vi "Teleop.vi"(8 "Driver Command Inputs":T8, 9 "Sensor Inputs":T1, 10 "Match Info":T16={"Autonomous Elapsed Seconds"=0.0, "TeleOp Elapsed Seconds"=0.0, "Disabled Elapsed Seconds"=0.0, "Visited Autonomous"=FALSE, "Visited TeleOp"=FALSE, "Visited Disabled"=FALSE, "Autonomous Settings"={"Autonomous Style"=enum."Independent", "VI Refnum"=refnum}}, 11 "Call Context":T17) -> (2 "Commands":T8, 3 "Sensor Inputs":T1)   [LabVIEW 2012]
doc: "This VI is called for each TeleOp packet received from the DS where the robot is not disabled. It is often used to read from the joysticks and update I/O or to update setpoints for timed control loops. It should complete and return within 20 milliseconds or it may miss DS packets."
uses:
  <vilib>/Rock Robotics/WPI/DriverStation/WPI_DriverStationDerivedRobotMode.ctl
  <vilib>/Rock Robotics/WPI/DriverStation/WPI_DriverStationMatch Info.ctl
  Inputs_All.ctl
  Flywheel/Sensor_Inputs_FlyWheel.ctl
  tankdrive/Input_Sensors_Drive.ctl
  Conveyor/Sensor_Input_Conveyor.ctl
  Conveyor/Sensor_Input_ConveyorV2.ctl
  Turret/Inputs_Sensors_Turret.ctl
  Inputs_Camera.ctl
  Command_Inputs.ctl
  tankdrive/Input_Commands_Drive.ctl
  Conveyor/Input_Command_Conveyor.ctl
  Turret/Inputs_Commands_Turret.ctl
  Bridge Tipper/Inputs_Tipper.ctl
  Dashboard Controls.ctl
  Roller/Input_Commands_Roller.ctl
  Flywheel/Input_Commands_Flywheel.ctl
  Robot Global Data.vi
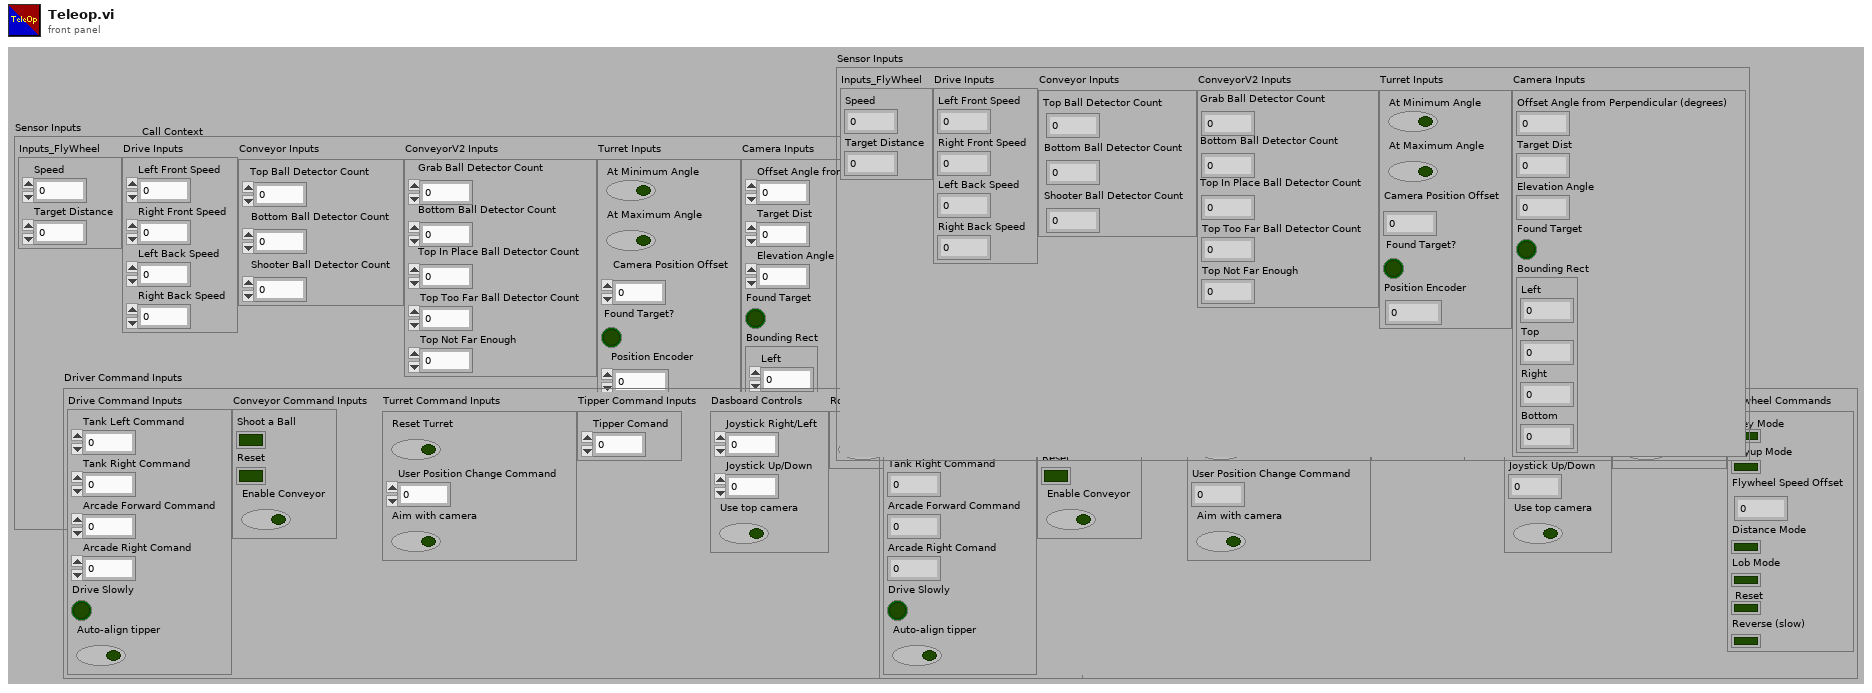
[diagram p1: front panel]
types:
  T1 = typedef "Inputs_All.ctl" = cluster{"Inputs_FlyWheel":T2, "Drive Inputs":T3, "Conveyor Inputs":T4, "ConveyorV2 Inputs":T5, "Turret Inputs":T6, "Camera Inputs":T7}
  T2 = typedef "Sensor_Inputs_FlyWheel.ctl" = cluster{"Speed":dbl, "Target Distance":dbl}
  T3 = typedef "Input_Sensors_Drive.ctl" = cluster{"Left Front Speed":dbl, "Right Front Speed":dbl, "Left Back Speed":dbl, "Right Back Speed":dbl}
  T4 = typedef "Sensor_Input_Conveyor.ctl" = cluster{"Top Ball Detector Count":i32, "Bottom Ball Detector Count":i32, "Shooter Ball Detector Count":i32}
  T5 = typedef "Sensor_Input_ConveyorV2.ctl" = cluster{"Grab Ball Detector Count":i32, "Bottom Ball Detector Count":i32, "Top In Place Ball Detector Count":i32, "Top Too Far Ball Detector Count":i32, "Top Not Far Enough":i32}
  T6 = typedef "Inputs_Sensors_Turret.ctl" = cluster{"At Minimum Angle":bool, "At Maximum Angle":bool, "Camera Position Offset":dbl, "Found Target?":bool, "Position Encoder":dbl}
  T7 = typedef "Inputs_Camera.ctl" = cluster{"Offset Angle from Perpendicular (degrees)":dbl, "Target Dist":dbl, "Elevation Angle":dbl, "Found Target":bool, "Bounding Rect":cluster{"Left":dbl, "Top":dbl, "Right":dbl, "Bottom":dbl}}
  T8 = typedef "Command_Inputs.ctl" = cluster{"Drive Command Inputs":T9, "Conveyor Command Inputs":T10, "Turret Command Inputs":T11, "Tipper Command Inputs":T12, "Dasboard Controls":T13, "Roller Commands":T14, "Flywheel Commands":T15}
  T9 = typedef "Input_Commands_Drive.ctl" = cluster{"Tank Left Command":dbl, "Tank Right Command":dbl, "Arcade Forward Command":dbl, "Arcade Right Comand":dbl, "Drive Slowly":bool, "Auto-align tipper":bool}
  T10 = typedef "Input_Command_Conveyor.ctl" = cluster{"Shoot a Ball":bool, "Reset":bool, "Enable Conveyor":bool}
  T11 = typedef "Inputs_Commands_Turret.ctl" = cluster{"Reset Turret":bool, "User Position Change Command":dbl, "Aim with camera":bool}
  T12 = typedef "Inputs_Tipper.ctl" = cluster{"Tipper Comand":dbl}
  T13 = typedef "Dashboard Controls.ctl" = cluster{"Joystick Right/Left":dbl, "Joystick Up/Down":dbl, "Use top camera":bool}
  T14 = typedef "Input_Commands_Roller.ctl" = cluster{"Enable Front Roller":bool}
  T15 = typedef "Input_Commands_Flywheel.ctl" = cluster{"Key Mode":bool, "Layup Mode":bool, "Flywheel Speed Offset":dbl, "Distance Mode":bool, "Lob Mode":bool, "Reset":bool, "Reverse (slow)":bool}
  T16 = typedef "WPI_DriverStationMatch Info.ctl" = cluster{"Autonomous Elapsed Seconds":dbl, "TeleOp Elapsed Seconds":dbl, "Disabled Elapsed Seconds":dbl, "Visited Autonomous":bool, "Visited TeleOp":bool, "Visited Disabled":bool, "Autonomous Settings":cluster{"Autonomous Style":enum16{"Iterative", "Independent"}, "VI Refnum":refnum<vi>}}
  T17 = typedef "WPI_DriverStationDerivedRobotMode.ctl" = enum16{"Init", "Execute", "Stop"}
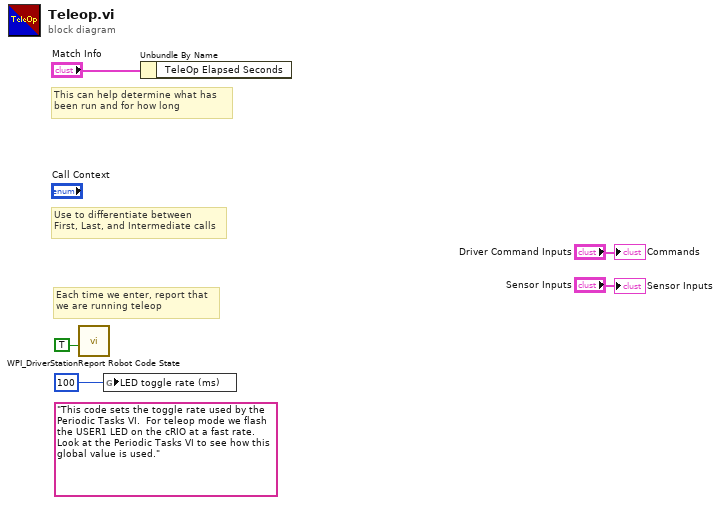
[diagram p0: block diagram]
diagram:
  (unwired) "This code sets the toggle rate used by the Periodic Tasks VI.  For teleop mode we flash the USER1 LED on the cRIO at a fast rate.  Look at the Periodic Tasks VI to see how this global value is used."
  # "Each time we enter, report that\nwe are running teleop"
  # "Use to differentiate between\nFirst, Last, and Intermediate calls"
  # "This can help determine what has\nbeen run and for how long"
  n1 = call <vilib>:"WPI_DriverStationReport Robot Code State.vi"("TeleOp"=TRUE ("Autonomous")) -> ()  [unwired: 10 in, 1 out]
  n2 = global write "Robot Global Data.vi" "LED toggle rate (ms)"(u32 100 ("LED ms toggle rate")) -> ()
  n3 = Unbundle By Name("Match Info") -> ()  [unwired: 1 out]
  "Commands" <- "Driver Command Inputs"
  "Sensor Inputs" <- "Sensor Inputs"
